vi "多参数关键参数读取.vi"(8 "Error in":errorcluster caption="Error in (no error)") -> (0 "error out":errorcluster, 3 "添加的数组":string[][](array[string]))   [LabVIEW 2016, in "斯坦道原位多参数.lvlib"]
panel:
  in  "关键参数区":i32(listbox)
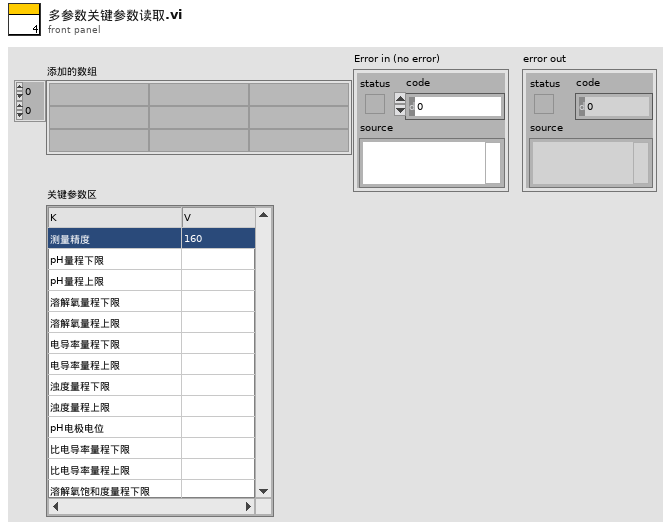
[diagram p1: front panel]
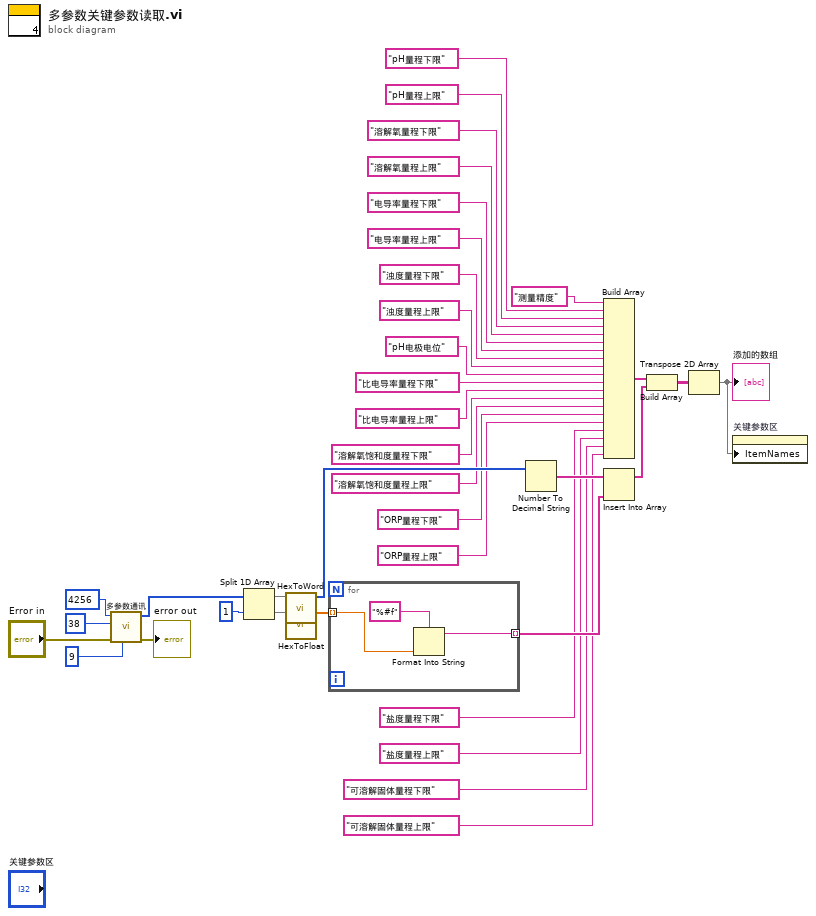
[diagram p0: block diagram]
diagram:
  n1 = call "多参数通讯.vi"("Slave ID"=u8 9, "Error in"="Error in", "quantity"=u16 38, "starting address"=u16 4256) -> ("error out"=→"error out":errorcluster, "Registers"=w35:u16[])  [unwired: 5 in, 1 out]
  n2 = Split 1D Array(array=w35, index=1 ("索引")) -> (first subarray=w21:u16[], second subarray=w20:u16[])
  n3 = call "HexToWord.vi"("数组"=w21) -> ("WORD"=w15:u16[])  [unwired: 10 in]
  n4 = call "HexToFloat.vi"("数组"=w20) -> ("FLOAT"=w13:sgl[])  [unwired: 10 in]
  n5 = for {
    tunnel: w13 -> [w39] mode=indexing
    tunnel: [w38] -> w12 mode=indexing
    n6 = Format Into String(format string="%#f" ("格式字符串"), w39) -> (resulting string=w38:string)  [unwired: 2 in, 1 out]
  }
  n7 = Number To Decimal String(number=w15) -> (decimal integer string=w14:string[])  [unwired: 1 in]
  n8 = Build Array("测量精度", "pH量程下限", "pH量程上限", "溶解氧量程下限", "溶解氧量程上限", "电导率量程下限", "电导率量程上限", "浊度量程下限", "浊度量程上限", "pH电极电位", "比电导率量程下限", "比电导率量程上限", "溶解氧饱和度量程下限", "溶解氧饱和度量程上限", "ORP量程下限", "ORP量程上限", "盐度量程下限", "盐度量程上限", "可溶解固体量程下限", "可溶解固体量程上限") -> (w23:string[])
  n9 = Insert Into Array(array=w14, new element=w12) -> (w19:string[])  [unwired: 1 in]
  n10 = Build Array(w23, w19) -> (w22:string[][])
  n11 = Transpose 2D Array(2D array=w22) -> (transposed array=w18:string[][])
  "添加的数组" <- w18
  n12 = property on="关键参数区" class="MCListbox (strict)"("ItemNames"=w18) -> ()  [unwired: 2 in, 2 out]
